vi "CAN UDS Response.vi"(6 "TimeOutMs":i32, 7 "pResData":u8[](array[numeric])=array[4097 elements], 9 "pUDSAddr":T1, 10 "CANIndex":u8, 11 "DevHandle":i32) -> (1 "pUDSAddr out":T1, 3 "function return":i32, 5 "pResData out":u8[](array[numeric]))   [LabVIEW 2010, in "can_uds.lvlib"]
doc: "int WINAPI CAN_UDS_Response(int DevHandle,unsigned char CANIndex,CAN_UDS_ADDR *pUDSAddr,unsigned char *pResData,int TimeOutMs);"
uses:
  can_uds.lvlib
  USB2XXX/trunk/USB2XXX/USB2XXX/vs2019/Release/USB2XXX.dll
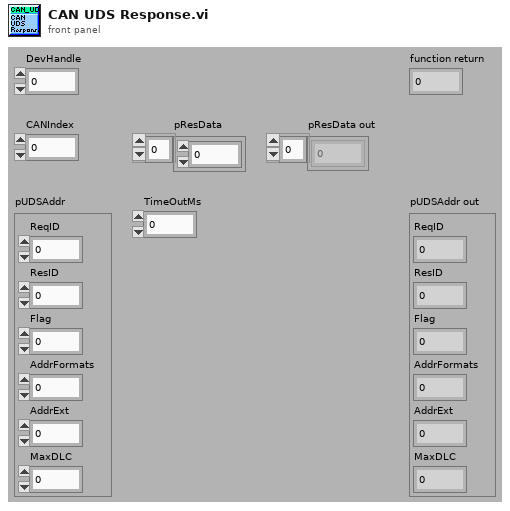
[diagram p1: front panel]
types:
  T1 = cluster{"ReqID":u32, "ResID":u32, "Flag":u8, "AddrFormats":u8, "AddrExt":u8, "MaxDLC":u8}
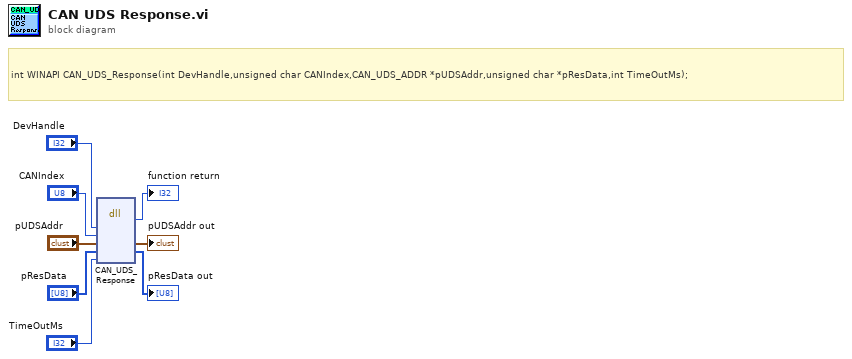
[diagram p0: block diagram]
diagram:
  # "int WINAPI CAN_UDS_Response(int DevHandle,unsigned char CANIndex,CAN_UDS_ADDR *pUDSAddr,unsigned char *pResData,int TimeOutMs);"
  n1 = dll-call lib="E:/Projects/USB2XXX/trunk/USB2XXX/USB2XXX/vs2019/Release/USB2XXX.*" fn="CAN_UDS_Response"("DevHandle"="DevHandle", "CANIndex"="CANIndex", "pUDSAddr"="pUDSAddr", "pResData"="pResData", "TimeOutMs"="TimeOutMs") -> (→"function return":i32, "pUDSAddr"=→"pUDSAddr out":T1, "pResData"=→"pResData out":u8[])  [unwired: 6 in, 2 out]
